vi "LCD1602Strings.vi"(5 "Address":u8=62 format="%.0x", 7 "Bus":u8=1, 8 "error in (no error)":errorcluster, 9 "String 2":string, 10 "String":string, 11 "Port":refnum<visa-resource-name>="COM5") -> (0 "error out":errorcluster={"status"=FALSE, "code"=1073676294, "source"="VISA Read in CTI-Visa.lvlib:Read Response.vi->CTI-Visa.lvlib:Read Identity.vi->TestLCD.vi"}, 3 "VISA resource name":refnum<visa-resource-name>)   [LabVIEW 2024]
uses:
  637507b3-f725-4c30-8ac4-b8c4abcf396b.vi
  680237c5-4512-48c9-a444-76735ded44a8.vi
  050e56bf-4e91-4887-a68b-f382978ec6c2.vi
  78847215-bff2-4261-a0c1-4f0a739d938a.vi
  Driver/CTIPicoVISA.lvlib
panel:
  # "Input"
  # "Output"
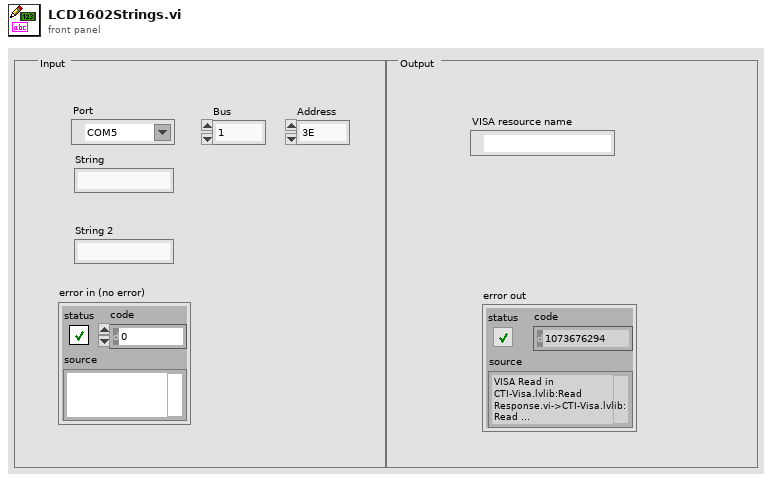
[diagram p1: front panel]
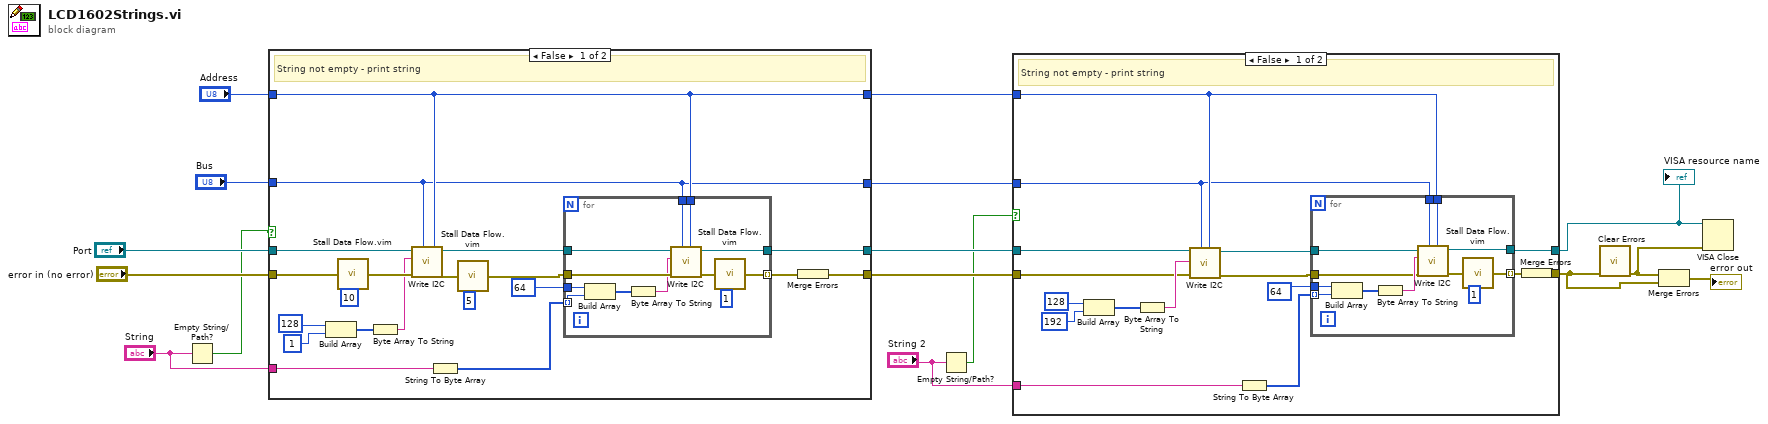
[diagram p0: block diagram]
diagram:
  n1 = Empty String/Path?(string/path="String") -> (empty?=w8:bool)
  n2 = case shown="False" w8 {
    tunnel: [w20 w51] -> w7
    tunnel: [w24 w52] -> w14
    tunnel: "Bus" -> [w17 w49]
    tunnel: "Address" -> [w18 w50]
    tunnel: "Port" -> [w23 w52]
    tunnel: "error in (no error)" -> [w22 w51]
    tunnel: "String" -> [w19 _]
    tunnel: [w18 w50] -> w4
    tunnel: [w17 w49] -> w3
    frame False {
      # "String not empty - print string"
      n3 = Build Array(u8 128 ("Value"), u8 1 ("Value")) -> (w32:u8[])
      n4 = call "Stall Data Flow.vim"("value in"=w22, "milliseconds to wait"=u32 10) -> ("value out"=w35:errorcluster)  [unwired: 1 out]
      n5 = Byte Array To String(unsigned byte array=w32) -> (string=w30:string)
      n6 = call "Write I2C.vi"("Address"=w18, "Bus"=w17, "error in (no error)"=w35, "Data"=w30, "VISA resource name in"=w23) -> ("error out"=w27:errorcluster, "VISA resource name"=w34:refnum<visa-resource-name>)  [unwired: 5 in]
      n7 = String To Byte Array(string=w19) -> (unsigned byte array=w33:u8[])
      n8 = call "Stall Data Flow.vim"("value in"=w27, "milliseconds to wait"=u32 5) -> ("value out"=w26:errorcluster)  [unwired: 1 out]
      n9 = for {
        tunnel: w34 -> [w48]
        tunnel: w26 -> [w47]
        tunnel: w17 -> [w46]
        tunnel: w18 -> [w45]
        tunnel: [w37] -> w21 mode=indexing
        tunnel: [w44] -> w24
        tunnel: w33 -> [w42] mode=indexing
        tunnel: u8 64 ("Value") -> [w41]
        n10 = Build Array(w41, w42) -> (w43:u8[])
        n11 = Byte Array To String(unsigned byte array=w43) -> (string=w40:string)
        n12 = call "Write I2C.vi"("Address"=w45, "Bus"=w46, "error in (no error)"=w47, "Data"=w40, "VISA resource name in"=w48) -> ("error out"=w38:errorcluster, "VISA resource name"=w44:refnum<visa-resource-name>)  [unwired: 5 in]
        n13 = call "Stall Data Flow.vim"("value in"=w38, "milliseconds to wait"=u32 1) -> ("value out"=w37:errorcluster)  [unwired: 1 out]
      }
      n14 = Merge Errors(w21) -> (w20:errorcluster)
    }
    frame True {
      # "String empty - so ignore"
    }
  }
  n15 = Empty String/Path?(string/path="String 2") -> (empty?=w2:bool)
  n16 = case shown="False" w2 {
    tunnel: w14 -> [w65 w82]
    tunnel: [w58 w82] -> w10
    tunnel: [w57 w81] -> w9
    tunnel: w7 -> [w56 w81]
    tunnel: w4 -> [w55 _]
    tunnel: w3 -> [w54 _]
    tunnel: "String 2" -> [w53 _]
    frame False {
      # "String not empty - print string"
      n17 = Build Array(u8 128 ("Value"), u8 192 ("Value")) -> (w60:u8[])
      n18 = Byte Array To String(unsigned byte array=w60) -> (string=w59:string)
      n19 = call "Write I2C.vi"("Address"=w55, "Bus"=w54, "error in (no error)"=w56, "Data"=w59, "VISA resource name in"=w65) -> ("error out"=w64:errorcluster, "VISA resource name"=w63:refnum<visa-resource-name>)  [unwired: 5 in]
      n20 = String To Byte Array(string=w53) -> (unsigned byte array=w67:u8[])
      n21 = for {
        tunnel: w54 -> [w80]
        tunnel: w55 -> [w79]
        tunnel: [w69] -> w68 mode=indexing
        tunnel: [w78] -> w58
        tunnel: w64 -> [w76]
        tunnel: w63 -> [w74]
        tunnel: w67 -> [w73] mode=indexing
        tunnel: u8 64 ("Value") -> [w72]
        n22 = Build Array(w72, w73) -> (w75:u8[])
        n23 = Byte Array To String(unsigned byte array=w75) -> (string=w77:string)
        n24 = call "Write I2C.vi"("Address"=w79, "Bus"=w80, "error in (no error)"=w76, "Data"=w77, "VISA resource name in"=w74) -> ("error out"=w70:errorcluster, "VISA resource name"=w78:refnum<visa-resource-name>)  [unwired: 5 in]
        n25 = call "Stall Data Flow.vim"("value in"=w70, "milliseconds to wait"=u32 1) -> ("value out"=w69:errorcluster)  [unwired: 1 out]
      }
      n26 = Merge Errors(w68) -> (w57:errorcluster)
    }
    frame True {
      # "String empty - so ignore"
    }
  }
  "VISA resource name" <- w10
  n27 = call <vilib>:"Clear Errors.vi"("error in (no error)"=w9) -> ("error out"=w15:errorcluster)  [unwired: 5 in, 1 out]
  n28 = Merge Errors(w15, w9) -> (→"error out":errorcluster)
  n29 = VISA Close(VISA resource name=w10, error in (no error)=w15) -> ()  [unwired: 1 out]
